vi "NI.AI_Points.vi"(0 "DAQmx设备名":tag="Dev2", 1 "input terminal configuration":i32(ring)=10106 caption="输入接线端配置" items=["默认"=-1, "RSE"=10083, "NRSE"=10078, "差分"=10106, "伪差分"=12529], 2 "Key-Freq":dbl min=0.0 step=0.1, 5 "AI Channel":T1(ring)=enum."AI3", 7 "Signal Filter":enum16{"None", "Low Pass", "High Pass"}(ring), 9 "SignalRate":u32=2500 caption="Samples" min=1, 11 "error in":errorcluster caption="错误输入", 12 "Rate":dbl=1.0) -> (3 "FREQ(Hz)":dbl=82736.97614753942, 4 "VPP(V)":dbl=0.006160413204242876, 6 "RMS(VDC)":dbl=0.6841750652888994, 10 "MAX(V)":dbl=0.6871733348618426, 13 "RMS(VAC)":dbl=0.0007020431731878134, 14 "波形图":waveform(dbl)(graph)={"t0"=timestamp(3513041668.599355 s since 1904-01-01), "dt"=3.999999999999989e-06, "Y"=array[2500 elements], "attributes"=variant("NI_ChannelName"=variant(string "Dev2/AI3"), "NI_UnitDescription"=variant(string "Volts"))}, 15 "error out":errorcluster caption="错误输出")   [LabVIEW 2012, in "Lib_UEL.ATE.lvlib" / "Lib_PCI6221.lvlib"]
uses:
  Lib_PCI6221.lvlib
  <vilib>/DAQmx/read.llb/DAQmx Read (Analog Wfm 1Chan NSamp).vi
  <vilib>/DAQmx/create/channels.llb/DAQmx Create Channel (AI-Voltage-Basic).vi
  <vilib>/DAQmx/configure/timing.llb/DAQmx Timing (Sample Clock).vi
  <vilib>/DAQmx/miscellaneous.llb/DAQmx Fill In Error Info.vi
panel:
  in  "测试日志信息 2":refnum<queue>
  # "V01 - Initial Version.  ~ LiGuang 2011-05-12\n        - Default, 波形图会显示四个周期 \nV02 - 2013/1/11, 增加日志功能: 将操作信息压入到输入的队列中.\nV03 - 2013/3/23, LiGuang, 增加Vrms(AC)计算,区分直流和交流有效值.\nV04 - 2015-4-28, LIGUANG, 增加滤波选项输出。滤波只针对AC波形及AC有效值。"
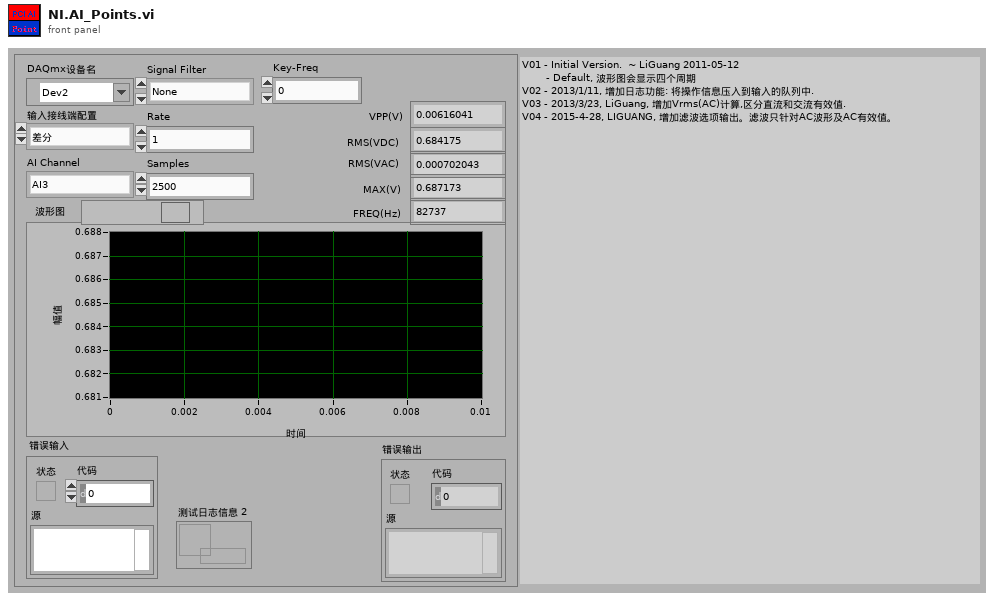
[diagram p1: front panel]
types:
  T1 = enum16{"AI0", "AI1", "AI2", "AI3", "AI4", "AI5", "AI6", "AI7", "AI8", "AI9", "AI10", "AI11", "AI12", "AI13", "AI14", "AI15"}
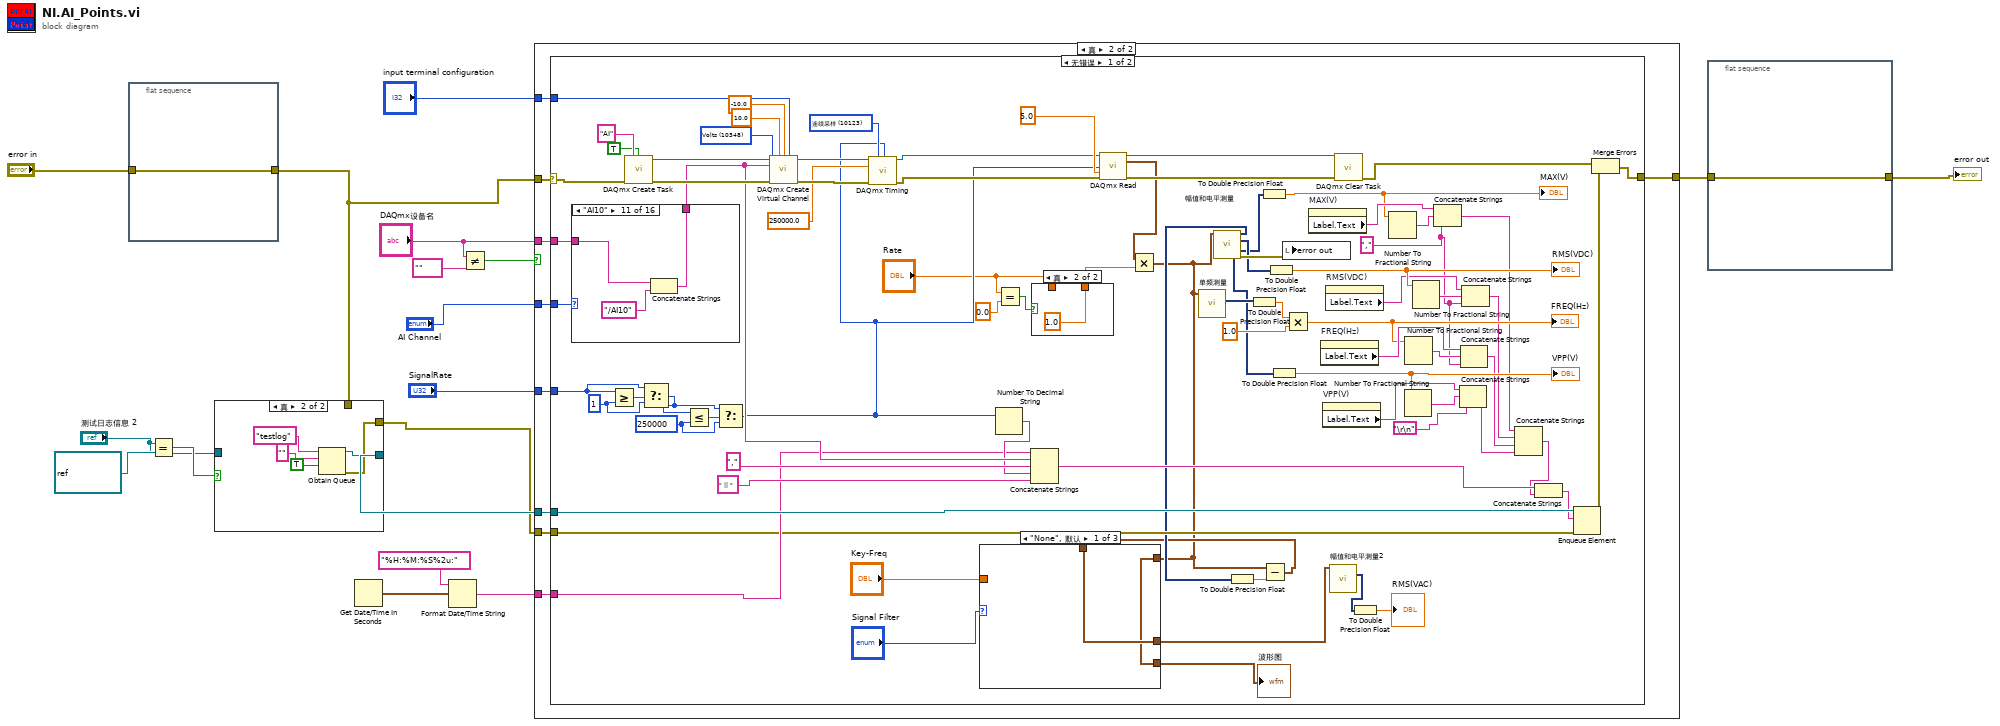
[diagram p0: block diagram]
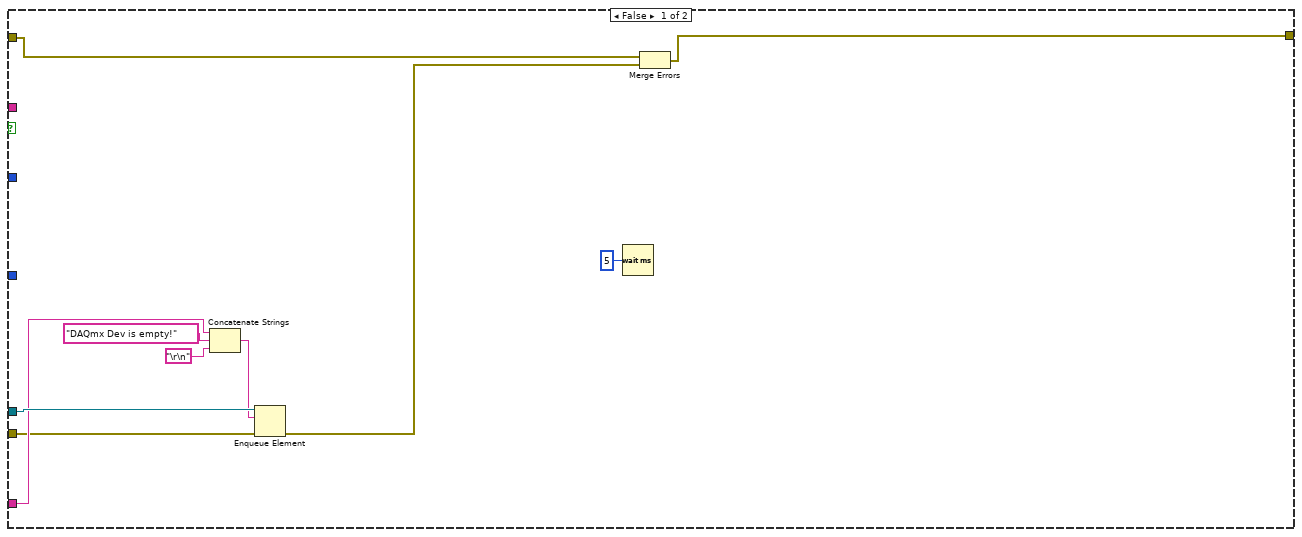
[diagram p3: hidden frame]
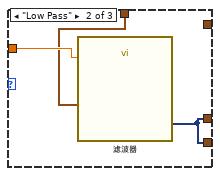
[diagram p4: hidden frame]
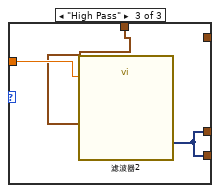
[diagram p5: hidden frame]
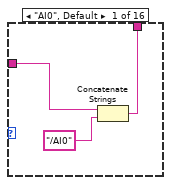
[diagram p7: hidden frame]
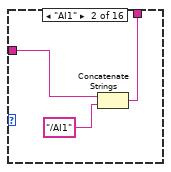
[diagram p8: hidden frame]
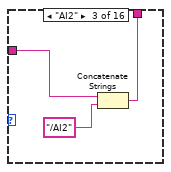
[diagram p9: hidden frame]
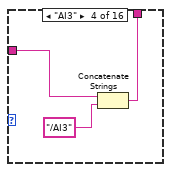
[diagram p10: hidden frame]
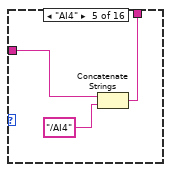
[diagram p11: hidden frame]
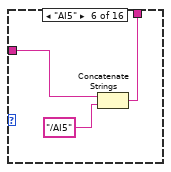
[diagram p12: hidden frame]
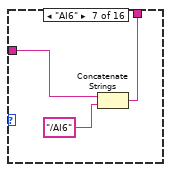
[diagram p13: hidden frame]
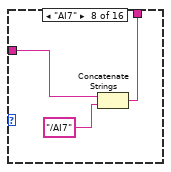
[diagram p14: hidden frame]
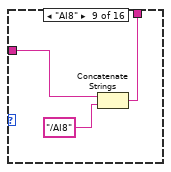
[diagram p15: hidden frame]
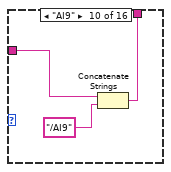
[diagram p16: hidden frame]
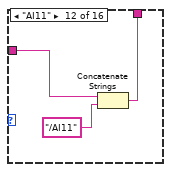
[diagram p17: hidden frame]
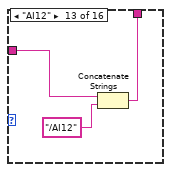
[diagram p18: hidden frame]
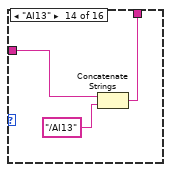
[diagram p19: hidden frame]
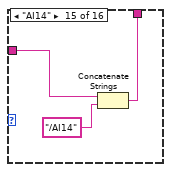
[diagram p20: hidden frame]
diagram:
  n1 = flat-sequence {
    tunnel: "error in" -> [w19]
    tunnel: [w19] -> w3
    frame #0 {
    }
  }
  n2 = Equal?(x="测试日志信息 2", y=refnum<queue> refnum ("测试日志信息")) -> (x = y?=w8:bool)
  n3 = case shown="真" w8 {
    tunnel: "测试日志信息 2" -> [w21 _]
    tunnel: [w21 w26] -> w6
    tunnel: [w20 w22] -> w5
    tunnel: w3 -> [w20 _]
    frame False {
    }
    frame True {
      n4 = Obtain Queue(name (unnamed)="testlog" ("名称（未命名）"), element data type="" ("名称（未命名）"), create if not found? (T)=TRUE ("如未找到是否创建？(T)")) -> (queue out=w26:refnum<queue>, error out=w22:errorcluster)  [unwired: 2 in, 1 out]
    }
  }
  n5 = Get Date/Time In Seconds() -> (seconds since 1Jan1904=w11:timestamp)
  n6 = Format Date/Time String(time format string (%c)="%H:%M:%S%2u:" ("时间格式化字符串(%c)"), seconds (now)=w11) -> (date/time string=w10:string)  [unwired: 1 in]
  n7 = Not Equal?(x="DAQmx设备名", y=tag "") -> (x != y?=w14:bool)
  n8 = case shown="真" w14 {
    tunnel: w3 -> [w31 w45]
    tunnel: [w29 w44] -> w2
    tunnel: "SignalRate" -> [_ w43]
    tunnel: "AI Channel" -> [_ w42]
    tunnel: "DAQmx设备名" -> [_ w41]
    tunnel: "input terminal configuration" -> [_ w40]
    tunnel: w6 -> [w36 w39]
    tunnel: w10 -> [w32 w38]
    tunnel: w5 -> [w27 w37]
    frame False {
      n9 = Concatenate Strings(w32, "DAQmx Dev is empty!" ("元素"), "\r\n") -> (w33:string)
      n10 = Enqueue Element(queue=w36, element=w33, error in (no error)=w27) -> (error out=w30:errorcluster)  [unwired: 1 in, 2 out]
      n11 = Wait (ms)(milliseconds to wait=u32 5 ("等待时间（毫秒）")) -> ()  [unwired: 1 out]
      n12 = Merge Errors(w31, w30) -> (w29:errorcluster)
    }
    frame True {
      n13 = case shown="无错误" w45 {
        selector: w45 -> [w125 w185]
        tunnel: [w101 w184] -> w44
        tunnel: w43 -> [w114 _]
        tunnel: w42 -> [w116 _]
        tunnel: w41 -> [w111 _]
        tunnel: w40 -> [w107 _]
        tunnel: w39 -> [w104 w190]
        tunnel: w38 -> [w76 w189]
        tunnel: w37 -> [w75 _]
        frame No Error {
          w67 = 10123 items=["有限采样"=10178, "连续采样"=10123, "硬件定时单点"=12522] ("sample mode")
          w70 = u32 250000 ("y")
          w113 = u32 1 ("y")
          w88 = "," ("时间格式化字符串(%c)")
          w119 = 10348 items=["Volts"=10348, "来自自定义换算"=10065] ("units")
          n14 = case shown="\"AI10\"" w116 {
            tunnel: [w136 w139 w142 w145 w148 w151 w154 w157 w160 w163 w166 w169 w172 w175 w178 w181] -> w100
            tunnel: w111 -> [w137 w140 w143 w146 w149 w152 w155 w158 w161 w164 w167 w170 w173 w176 w179 w182]
            frame "AI0", Default {
              n15 = Concatenate Strings(w137, "/AI0") -> (w136:string)
            }
            frame "AI1" {
              n16 = Concatenate Strings(w140, "/AI1") -> (w139:string)
            }
            frame "AI2" {
              n17 = Concatenate Strings(w143, "/AI2") -> (w142:string)
            }
            frame "AI3" {
              n18 = Concatenate Strings(w146, "/AI3") -> (w145:string)
            }
            frame "AI4" {
              n19 = Concatenate Strings(w149, "/AI4") -> (w148:string)
            }
            frame "AI5" {
              n20 = Concatenate Strings(w152, "/AI5") -> (w151:string)
            }
            frame "AI6" {
              n21 = Concatenate Strings(w155, "/AI6") -> (w154:string)
            }
            frame "AI7" {
              n22 = Concatenate Strings(w158, "/AI7") -> (w157:string)
            }
            frame "AI8" {
              n23 = Concatenate Strings(w161, "/AI8") -> (w160:string)
            }
            frame "AI9" {
              n24 = Concatenate Strings(w164, "/AI9") -> (w163:string)
            }
            frame "AI10" {
              n25 = Concatenate Strings(w167, "/AI10") -> (w166:string)
            }
            frame "AI11" {
              n26 = Concatenate Strings(w170, "/AI11") -> (w169:string)
            }
            frame "AI12" {
              n27 = Concatenate Strings(w173, "/AI12") -> (w172:string)
            }
            frame "AI13" {
              n28 = Concatenate Strings(w176, "/AI13") -> (w175:string)
            }
            frame "AI14" {
              n29 = Concatenate Strings(w179, "/AI14") -> (w178:string)
            }
            frame "AI15" {
              n30 = Concatenate Strings(w182, "/AI15") -> (w181:string)
            }
          }
          n31 = Greater Or Equal?(x=w114, y=w113) -> (x >= y?=w115:bool)
          n32 = call <vilib>:"DAQmx Create Task.vi"("new task name"="AI", "auto cleanup"=TRUE, "error in"=w125) -> ("task out"=w123:refnum<k21>, "error out"=w122:errorcluster)  [unwired: 11 in]
          n33 = Select(t=w114, s=w115, f=w113) -> (s? t:f=w68:u32)
          n34 = Less Or Equal?(x=w68, y=w70) -> (x <= y?=w69:bool)
          n35 = Select(t=w68, s=w69, f=w70) -> (s? t:f=w66:u32)
          n36 = call-poly <vilib>:"DAQmx Create Virtual Channel.vi"("task in"=w123, "maximum value"=10.0, "minimum value"=-10.0, "input terminal configuration"=w107, "physical channels"=w100, "units"=w119, "error in"=w122) -> ("task out"=w118:refnum<k21>, "error out"=w117:errorcluster)  [unwired: 7 in]
          n37 = call-poly <vilib>:"DAQmx Timing.vi"("task/channels in"=w118, "sample mode"=w67, "samples per channel"=w66, "rate"=250000.0, "error in"=w117) -> ("task out"=w72:refnum<k21>, "error out"=w71:errorcluster)  [unwired: 9 in]
          n38 = Number To Decimal String(number=w66) -> (decimal integer string=w98:string)  [unwired: 1 in]
          n39 = Equal?(x="Rate", y=0.0) -> (x = y?=w61:bool)
          n40 = Concatenate Strings(w76, w100, "," ("时间格式化字符串(%c)"), w98, " || " ("时间格式化字符串(%c)")) -> (w79:string)
          n41 = case shown="真" w61 {
            tunnel: [w134 1.0 ("rate")] -> w60
            tunnel: "Rate" -> [w134 _]
            frame False {
            }
            frame True {
            }
          }
          n42 = call-poly <vilib>:"DAQmx Read.vi"("task/channels in"=w72, "number of samples per channel"=w66, "timeout"=5.0, "error in"=w71) -> ("task out"=w121:refnum<k21>, "data"=w62:waveform(dbl), "error out"=w120:errorcluster)  [unwired: 9 in]
          n43 = Multiply(x=w62, y=w60) -> (x*y=w46:waveform(dbl))
          n44 = call "单频测量"("Signals"=w46) -> ("Frequency"=w65:dynamicdata)  [unwired: 8 in, 2 out]
          n45 = call "幅值和电平测量"("Signals"=w46) -> ("Mean (DC)"=w51:dynamicdata, "RMS"=w56:dynamicdata, "Positive Peak"=w55:dynamicdata, "Peak to Peak"=w54:dynamicdata, "error out"=w64:errorcluster)  [unwired: 10 in]
          n46 = To Double Precision Float(number=w51) -> (double precision float=w57:dbl)
          n47 = To Double Precision Float(number=w65) -> (double precision float=w110:dbl)
          n48 = To Double Precision Float(number=w55) -> (double precision float=w73:dbl)
          "MAX(V)" <- w73
          n49 = Subtract(x=w46, y=w57) -> (x-y=w50:waveform(dbl))
          n50 = case shown="\"None\", 默认" "Signal Filter" {
            tunnel: w50 -> [w127 w129 w132]
            tunnel: "Key-Freq" -> [_ w130 w133]
            tunnel: [w127 w128 w131] -> w48
            tunnel: [w126 w128 w131] -> w47
            tunnel: w46 -> [w126 _ _]
            frame "None", Default {
            }
            frame "Low Pass" {
              n51 = call "滤波器"("Lower Cut-Off"=w130, "Signal"=w129) -> ("Filtered Signal"=w128:dynamicdata)  [unwired: 8 in, 1 out]
            }
            frame "High Pass" {
              n52 = call "滤波器2"("Lower Cut-Off"=w133, "Signal"=w132) -> ("Filtered Signal"=w131:dynamicdata)  [unwired: 8 in, 1 out]
            }
          }
          "波形图" <- w47
          n53 = To Double Precision Float(number=w56) -> (double precision float=w94:dbl)
          "RMS(VDC)" <- w94
          n54 = To Double Precision Float(number=w54) -> (double precision float=w87:dbl)
          "VPP(V)" <- w87
          n55 = local write "error out"(w64) -> ()
          n56 = Multiply(x=w110, y=1.0 ("rate")) -> (x*y=w89:dbl)
          "FREQ(Hz)" <- w89
          n57 = property on="MAX(V)" class="DigNum (严格)"() -> ("Label.Text"=w96:string)  [unwired: 2 in, 2 out]
          n58 = property on="FREQ(Hz)" class="DigNum (严格)"() -> ("Label.Text"=w91:string)  [unwired: 2 in, 2 out]
          n59 = property on="VPP(V)" class="DigNum (严格)"() -> ("Label.Text"=w86:string)  [unwired: 2 in, 2 out]
          n60 = property on="RMS(VDC)" class="DigNum (严格)"() -> ("Label.Text"=w93:string)  [unwired: 2 in, 2 out]
          n61 = call "幅值和电平测量2"("Signals"=w48) -> ("RMS"=w49:dynamicdata)  [unwired: 13 in, 1 out]
          n62 = call <vilib>:"DAQmx Clear Task.vi"("task in"=w121, "error in"=w120) -> ("error out"=w103:errorcluster)  [unwired: 13 in]
          n63 = To Double Precision Float(number=w49) -> (double precision float=→"RMS(VAC)":dbl)
          n64 = Number To Fractional String(number=w73) -> (F-format string=w95:string)  [unwired: 3 in]
          n65 = Number To Fractional String(number=w87) -> (F-format string=w85:string)  [unwired: 3 in]
          n66 = Number To Fractional String(number=w89) -> (F-format string=w90:string)  [unwired: 3 in]
          n67 = Number To Fractional String(number=w94) -> (F-format string=w92:string)  [unwired: 3 in]
          n68 = Concatenate Strings(w96, w95, w88) -> (w83:string)
          n69 = Concatenate Strings(w86, w85, "\r\n") -> (w80:string)
          n70 = Concatenate Strings(w91, w90, w88) -> (w81:string)
          n71 = Concatenate Strings(w93, w92, w88) -> (w82:string)
          n72 = Concatenate Strings(w83, w82, w81, w80) -> (w78:string)
          n73 = Concatenate Strings(w79, w78) -> (w77:string)
          n74 = Enqueue Element(queue=w104, element=w77, error in (no error)=w75) -> (error out=w102:errorcluster)  [unwired: 1 in, 2 out]
          n75 = Merge Errors(w103, w102) -> (w101:errorcluster)
        }
        frame Error {
          n76 = Wait (ms)(milliseconds to wait=u32 5 ("等待时间（毫秒）")) -> ()  [unwired: 1 out]
          n77 = Concatenate Strings(w189, "Some ERR input." ("元素"), "\r\n") -> (w191:string)
          n78 = Enqueue Element(queue=w190, element=w191, error in (no error)=errorcluster {"status"=FALSE, "code"=0, "source"=""} ("错误输入（无错误）")) -> (error out=w186:errorcluster)  [unwired: 1 in, 2 out]
          n79 = Merge Errors(w185, w186) -> (w184:errorcluster)
        }
      }
    }
  }
  n80 = flat-sequence {
    tunnel: w2 -> [w194]
    tunnel: [w194] -> w1
    frame #0 {
    }
  }
  "error out" <- w1
